vi "MARS Update Scan Data Channels.vi"(11 "Listbox":i32[](array[numeric])) -> ()   [LabVIEW 2015]
uses:
  Data_Analysis_subvis/ESA_Data_Analysis_Global_VIs.vi
  Data_Analysis_subvis/MARS_Scan_Data_Analysis_global.vi
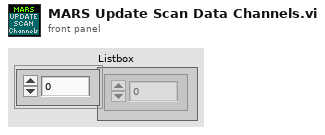
[diagram p1: front panel]
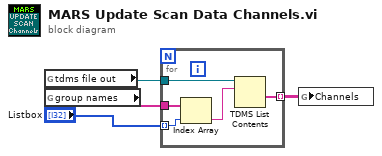
[diagram p0: block diagram]
diagram:
  n1 = global read "ESA_Data_Analysis_Global_VIs.vi" "tdms file out"() -> (w1:refnum<k34>)
  n2 = global read "ESA_Data_Analysis_Global_VIs.vi" "group names"() -> (w2:string[])
  n3 = for {
    tunnel: w1 -> [w7]
    tunnel: "Listbox" -> [w8] mode=indexing
    tunnel: w2 -> [w9]
    tunnel: [w5] -> w3 mode=indexing
    n4 = Index Array(array=w9, index=w8) -> (element=w6:string)
    n5 = TDMS List Contents(6:w6, 7:w7) -> (1:w5:string[])  [unwired: 1 in, 3 out]
  }
  n6 = global write "MARS_Scan_Data_Analysis_global.vi" "Channels"(w3) -> ()
